vi "4Pi Obj Lock - Rotate Flip XY.vi"(0 "XY Amounts":dbl[](array[numeric]), 7 "Flip XY":bool, 9 "Invert X":bool, 11 "Invert Y":bool) -> (4 "45° Rotated XY":dbl[](array[numeric]))   [LabVIEW 2016]
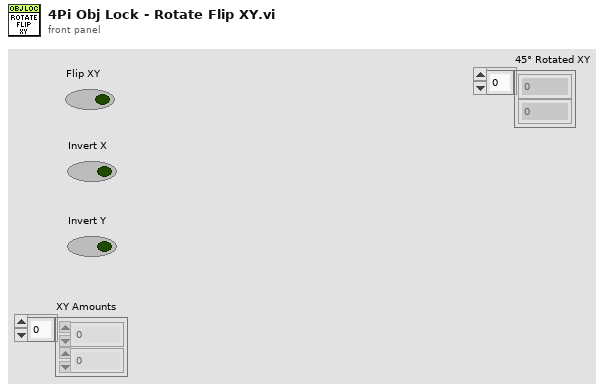
[diagram p1: front panel]
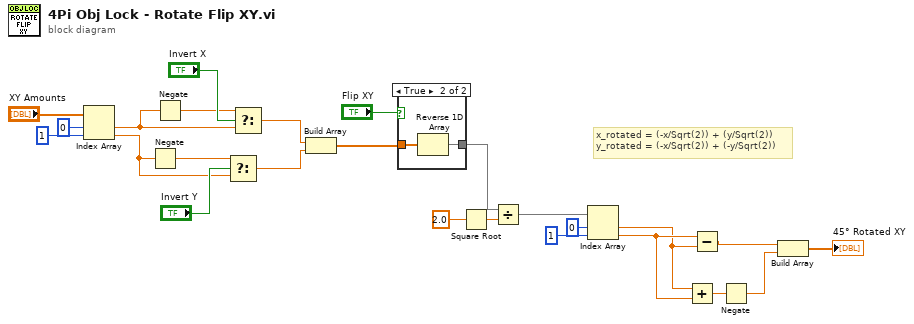
[diagram p0: block diagram]
diagram:
  # "x_rotated = (-x/Sqrt(2)) + (y/Sqrt(2))\ny_rotated = (-x/Sqrt(2)) + (-y/Sqrt(2))"
  n1 = Index Array(array="XY Amounts", index #1=0 ("index"), index #2=1 ("index")) -> (element #1=w12:dbl, element #2=w9:dbl)
  n2 = Negate(x=w9) -> (-x=w11:dbl)
  n3 = Negate(x=w12) -> (-x=w13:dbl)
  n4 = Select(t=w11, s="Invert Y", f=w9) -> (s? t:f=w7:dbl)
  n5 = Select(t=w13, s="Invert X", f=w12) -> (s? t:f=w8:dbl)
  n6 = Build Array(w8, w7) -> (w5:dbl[])
  n7 = case shown="True" "Flip XY" {
    tunnel: w5 -> [w26 w28]
    tunnel: [w26 w27] -> w4
    frame False {
    }
    frame True {
      n8 = Reverse 1D Array(array=w28) -> (reversed array=w27:dbl[])
    }
  }
  n9 = Square Root(x=2.0) -> (sqrt(x)=w21:dbl)
  n10 = Divide(x=w4, y=w21) -> (x/y=w20:dbl[])
  n11 = Index Array(array=w20, index #1=0 ("index"), index #2=1 ("index")) -> (element #1=w18:dbl, element #2=w19:dbl)
  n12 = Add(x=w18, y=w19) -> (x+y=w22:dbl)
  n13 = Subtract(x=w19, y=w18) -> (x-y=w2:dbl)
  n14 = Negate(x=w22) -> (-x=w1:dbl)
  n15 = Build Array(w2, w1) -> (→"45° Rotated XY":dbl[])
